vi "DataPacker_MainStateMachine.vi"(0 "DataPacker Queue":refnum<queue>, 1 "DataPacker out":refnum<class "DataPacker.lvclass">, 2 "error IO":errorcluster, 3 "Callers (Main VI name)":string, 6 "MIDAS IP":u32, 8 "MIDAS Sever Port":u16, 10 "Override Max Event size (Data rate bytes/s). Use MIDAS Default = 0":u32) -> (16 "error IO 2":errorcluster)   [LabVIEW 2018, in "feGEM DataPacker.lvlib"]
uses:
  feGEM DataPacker.lvlib
  DataStructures/GEM_BANK_CLUSTER_typedef.ctl
  DataStructures/GEM_DATA_cluster_typedef.ctl
  DataPacker.lvclass
  StateMachineTypeDef.ctl
  GlobalVariables/DataPacker_Global_Stop_Enum.ctl
  DataPacker.lvclass/DataPacker.ctl
  GlobalVariables/DataPacker_Buffer_Usage_Enum.ctl
  GlobalVariables/Set_And_Get_Enum.ctl
  <vilib>/Utility/SystemLogging/NI_SystemLogging.lvlib
panel:
  out "Time since last sleep (ms) 2":dbl(knob) scale=1.0..1000.0
  out "Time Bundling Data (Reading from Queue into LV structures) 2":dbl(knob) scale=0.0..100.0
  out "% Time Packing (Serializing Queued Data) 2":dbl(knob) scale=0.0..100.0
  out "Unsent items in queue (at shutdown)":i32
  out "Frontend Status":string
  out "MIDAS Port":u16
  out "MIDAS Addresss":string
  out "Connection Attempt":u32
  out "MIDAS Reply":string
  out "MIDAS Buffer [for this PC] \nUsage (%)":dbl(knob) scale=0.0..100.0
  out "Log Client info (non fatal)":errorcluster
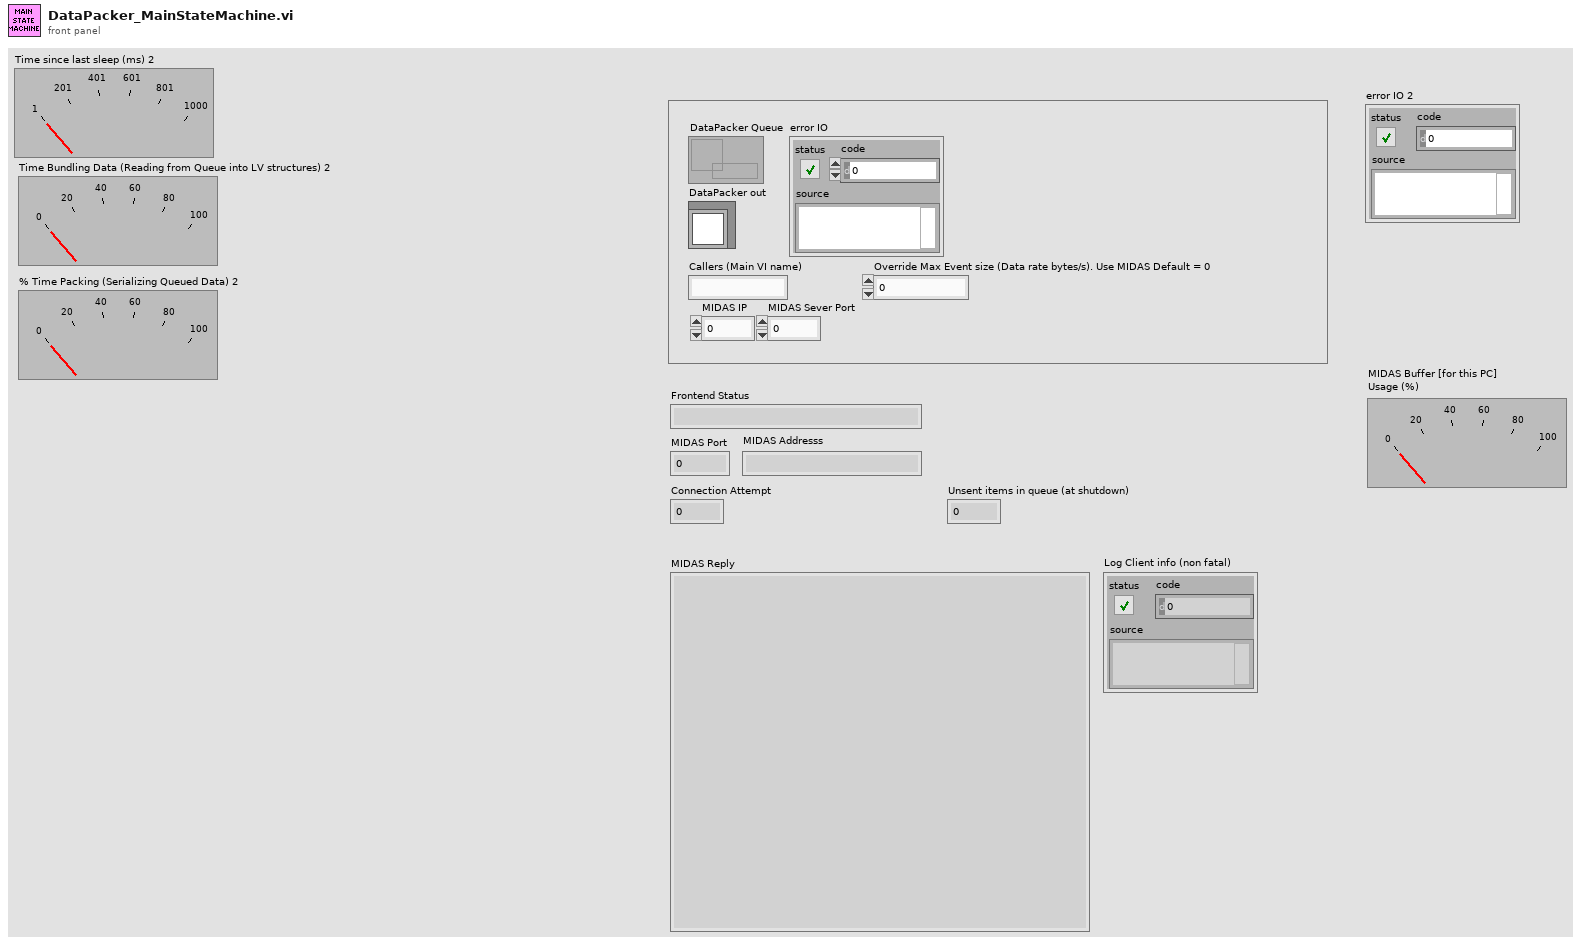
[diagram p1: front panel]
types:
  T1 = typedef "feGEM DataPacker.lvlib/StateMachineTypeDef.ctl" = enum16{"Setup", "Setup SSH", "Connect To Midas", "Get And Set Event Size", "Re-initialise", "Update status", "BundleDataInQueue", "SerializeBundle", "SendData", "Shutdown", "HandleErrorStates", "Wait"}
  T2 = typedef "feGEM DataPacker.lvlib/DataPacker_Global_Stop_Enum.ctl" = enum16{"Reset", "Set Soft Stop", "Get Soft Stop", "Set Hard Stop", "Get Hard Stop", "Get Any Stop"}
  T3 = typedef "feGEM DataPacker.lvlib/DataPacker_Buffer_Usage_Enum.ctl" = enum16{"Get Values", "Set MIDAS Buffer Usage (%)", "Set DataPacker Queue\nUsage (%)"}
  T4 = typedef "feGEM DataPacker.lvlib/Set_And_Get_Enum.ctl" = enum16{"Set", "Get"}
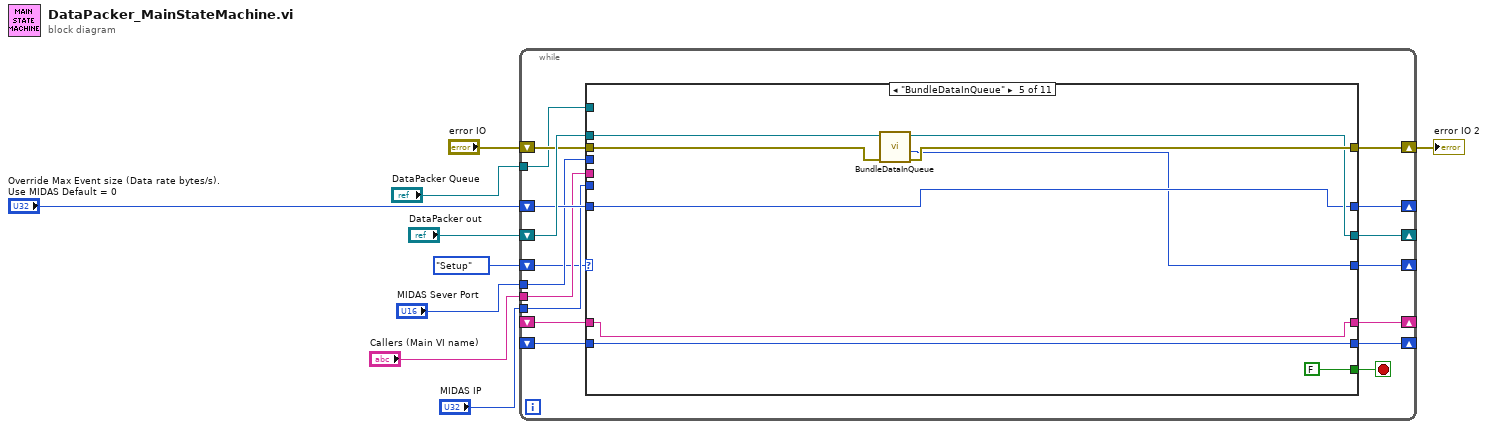
[diagram p0: block diagram]
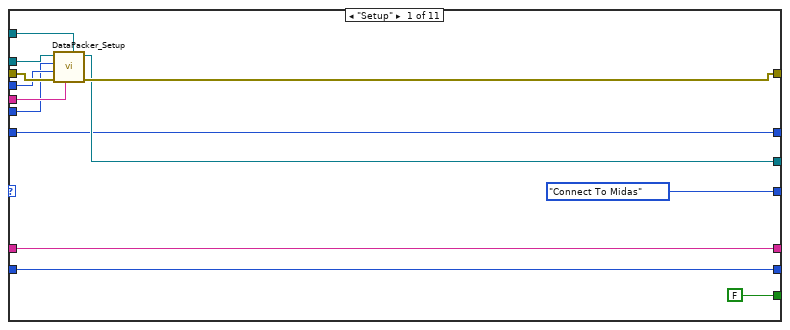
[diagram p2: hidden frame]
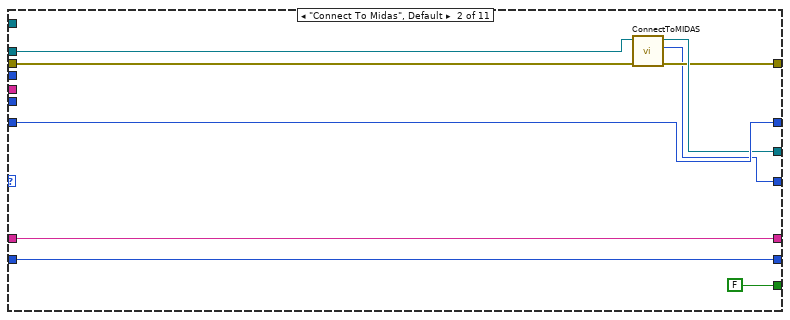
[diagram p3: hidden frame]
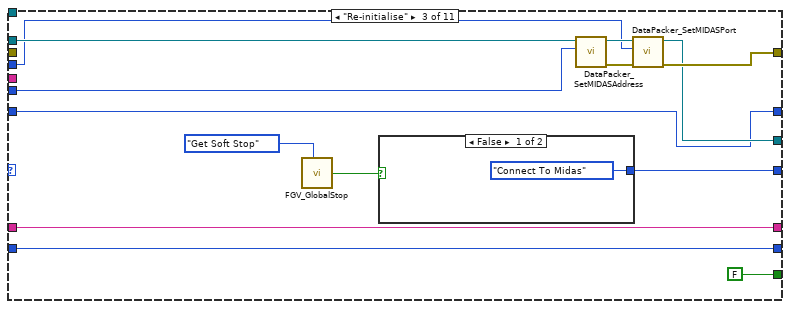
[diagram p4: hidden frame]
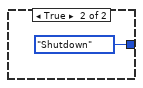
[diagram p5: hidden frame]
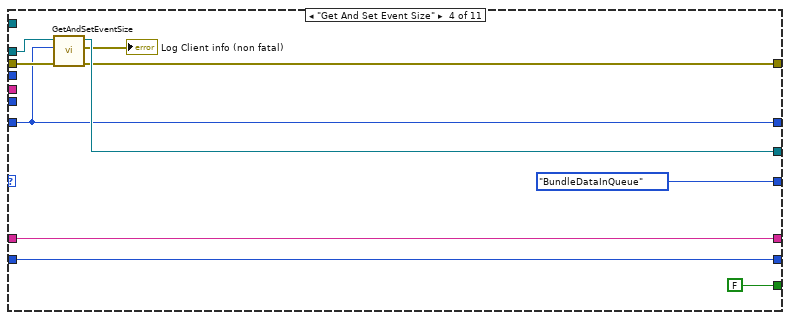
[diagram p6: hidden frame]
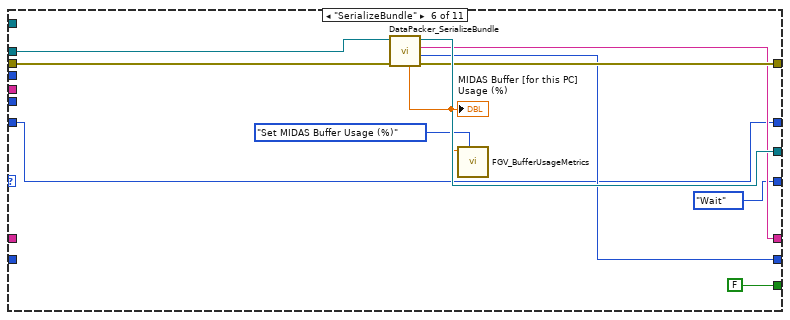
[diagram p7: hidden frame]
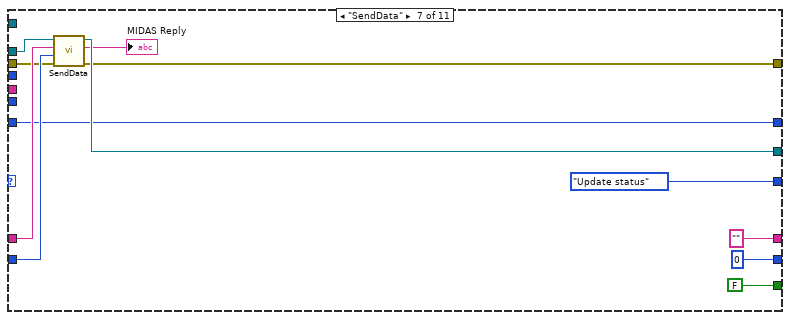
[diagram p8: hidden frame]
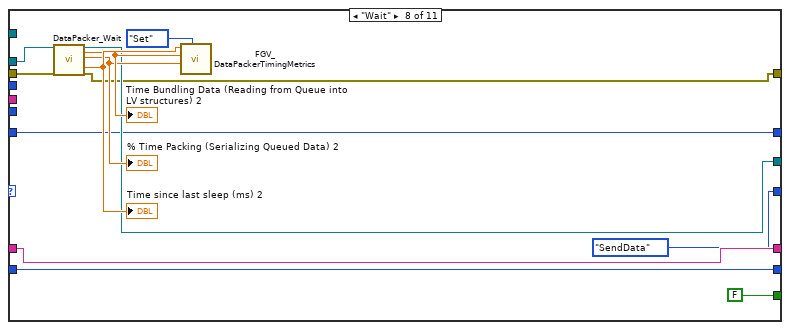
[diagram p9: hidden frame]
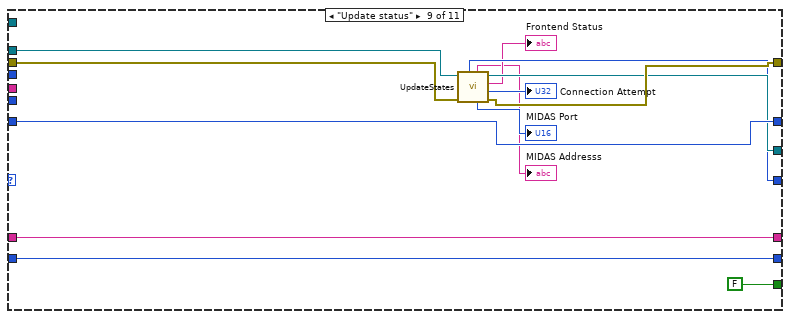
[diagram p10: hidden frame]
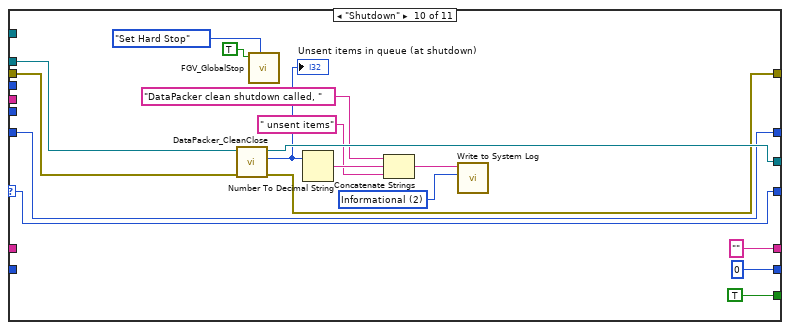
[diagram p11: hidden frame]
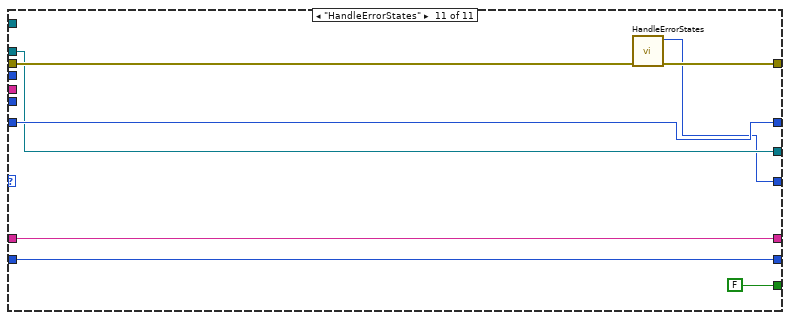
[diagram p12: hidden frame]
diagram:
  n1 = while {
    shift-right: [w10] -> _
    shift-left: StateMachineTypeDef."Setup" ("Enum") -> [w11]
    shift-right: [w24] -> _
    shift-left: "DataPacker out" -> [w26]
    shift-right: [w23] -> w1
    shift-left: "error IO" -> [w25]
    shift-right: [w21] -> _
    shift-left: _ -> [w18]
    shift-right: [w20] -> _
    shift-left: _ -> [w19]
    shift-right: [w17] -> _
    shift-left: "Override Max Event size (Data rate bytes/s). Use MIDAS Default = 0" -> [w22]
    tunnel: "MIDAS Sever Port" -> [w16]
    tunnel: "Callers (Main VI name)" -> [w15]
    tunnel: "DataPacker Queue" -> [w13]
    tunnel: "MIDAS IP" -> [w12]
    stop <- w14 stop-if-true
    n2 = case shown="\"BundleDataInQueue\"" w11 {
      selector: w11 -> [_ _ _ _ _ _ _ _ _ w133 _]
      tunnel: w26 -> [w37 w48 w58 w74 w83 w94 w97 w115 w132 w149 w152]
      tunnel: w25 -> [w39 w47 _ w73 w76 w93 w96 w113 w131 w147 w157]
      tunnel: [w35 w42 w59 w72 w81 w92 w104 w114 w125 w148 w152] -> w24
      tunnel: [w36 w41 w60 w67 w82 w91 w99 w112 w126 w134 w156] -> w23
      tunnel: w22 -> [w33 w44 w53 w68 w77 w87 w100 w109 w127 w143 w155]
      tunnel: [w31 w45 w55 w70 w79 w90 "" w111 w130 "" ("SerialisedData") w153] -> w21
      tunnel: [w32 w43 w54 w69 w80 w89 0 ("Length of \nData bundle") w110 w129 0 ("Length of \nData bundle") w154] -> w20
      tunnel: w19 -> [w32 w43 w54 w69 w80 _ w106 w110 w129 _ w154]
      tunnel: w18 -> [w31 w45 w55 w70 w79 _ w105 w111 w130 _ w153]
      tunnel: [FALSE FALSE FALSE FALSE FALSE FALSE FALSE FALSE FALSE TRUE FALSE] -> w14
      tunnel: [w33 w44 w53 w68 w77 w87 w100 w109 w127 w143 w155] -> w17
      tunnel: w16 -> [w38 _ w57 _ _ _ _ _ _ _ _]
      tunnel: w15 -> [w34 _ _ _ _ _ _ _ _ _ _]
      tunnel: w13 -> [w29 _ _ _ _ _ _ _ _ _ _]
      tunnel: w12 -> [w28 _ w56 _ _ _ _ _ _ _ _]
      tunnel: [StateMachineTypeDef."Connect To Midas" ("Enum") w40 w49 StateMachineTypeDef."BundleDataInQueue" ("Enum") w75 StateMachineTypeDef."Wait" ("Enum") StateMachineTypeDef."Update status" ("Enum") StateMachineTypeDef."SendData" ("Enum") w124 w133 w150] -> w10
      frame "Setup" {
        n3 = call "DataPacker_Setup.vi"("DataPacker Queue"=w29, "Main VI Name"=w34, "error in (no error)"=w39, "Port To Log To"=w38, "Address to Log To"=w28, "DataPacker in"=w37) -> ("error out"=w36:errorcluster, "DataPacker out"=w35:refnum<class "DataPacker.lvclass">)  [unwired: 4 in]
      }
      frame "Connect To Midas", Default {
        n4 = call "ConnectToMIDAS.vi"("error in (no error)"=w47, "DataPacker in"=w48) -> ("error out"=w41:errorcluster, "Enum"=w40:T1, "DataPacker out"=w42:refnum<class "DataPacker.lvclass">)  [unwired: 7 in]
      }
      frame "Re-initialise" {
        n5 = call "FGV_GlobalStop.vi"("Enum"=DataPacker_Global_Stop_Enum."Get Soft Stop") -> ("Stop"=w50:bool)  [unwired: 4 in]
        n6 = case shown="False" w50 {
          tunnel: [StateMachineTypeDef."Connect To Midas" ("Enum") StateMachineTypeDef."Shutdown" ("Enum")] -> w49
          frame False {
          }
          frame True {
          }
        }
        n7 = call "DataPacker_SetMIDASAddress.vi"("Address to Log To"=w56, "DataPacker in"=w58) -> ("error out"=w61:errorcluster, "DataPacker out"=w62:refnum<class "DataPacker.lvclass">)  [unwired: 8 in]
        n8 = call "DataPacker_SetMIDASPort.vi"("error in (no error)"=w61, "Port To Log To"=w57, "DataPacker in"=w62) -> ("error out"=w60:errorcluster, "DataPacker out"=w59:refnum<class "DataPacker.lvclass">)  [unwired: 7 in]
      }
      frame "Get And Set Event Size" {
        n9 = call "GetAndSetEventSize.vi"("error in (no error)"=w73, "Override Max Event size (Data rate bytes/s). Use MIDAS Default = 0"=w68, "DataPacker in"=w74) -> ("error out"=w67:errorcluster, "Log Client info (non fatal)"=→"Log Client info (non fatal)":errorcluster, "DataPacker out"=w72:refnum<class "DataPacker.lvclass">)  [unwired: 6 in]
      }
      frame "BundleDataInQueue" {
        n10 = call "BundleDataInQueue.vi"("error in (no error)"=w76, "DataPacker in"=w83) -> ("error out"=w82:errorcluster, "Enum"=w75:T1, "DataPacker out"=w81:refnum<class "DataPacker.lvclass">)  [unwired: 7 in]
      }
      frame "SerializeBundle" {
        n11 = call "DataPacker_SerializeBundle.vi"("error in (no error)"=w93, "DataPacker in"=w94) -> ("error out"=w91:errorcluster, "Length of \nData bundle"=w89:i32, "SerialisedData"=w90:string, "DataPacker out"=w92:refnum<class "DataPacker.lvclass">, "MIDAS Buffer \n[for this PC] \nUsage (%)"=w86:dbl)  [unwired: 5 in]
        "MIDAS Buffer [for this PC] \nUsage (%)" <- w86
        n12 = call "FGV_BufferUsageMetrics.vi"(7:DataPacker_Buffer_Usage_Enum."Set MIDAS Buffer Usage (%)", "Input"=w86) -> ()  [unwired: 8 in, 2 out]
      }
      frame "SendData" {
        n13 = call "SendData.vi"("error in (no error)"=w96, "Length of \nData bundle"=w106, "SerialisedData"=w105, "DataPacker in"=w97) -> ("error out"=w99:errorcluster, "MIDAS Reply"=→"MIDAS Reply":string, "DataPacker out"=w104:refnum<class "DataPacker.lvclass">)  [unwired: 5 in]
      }
      frame "Wait" {
        n14 = call "DataPacker_Wait.vi"("DataPacker in"=w115, "error in (no error)"=w113) -> ("DataPacker out"=w114:refnum<class "DataPacker.lvclass">, "% Time Bundling Data (Reading from Queue into LV structures)"=w118:dbl, "% Time Packing (Serializing Queued Data)"=w117:dbl, "Time since last sleep(ms)"=w119:dbl, "error out"=w112:errorcluster)  [unwired: 12 in, 1 out]
        "% Time Packing (Serializing Queued Data) 2" <- w117
        "Time Bundling Data (Reading from Queue into LV structures) 2" <- w118
        "Time since last sleep (ms) 2" <- w119
        n15 = call "FGV_DataPackerTimingMetrics.vi"(7:Set_And_Get_Enum."Set", "% Time Packing (Serializing Queued Data)"=w117, "Time Bundling Data (Reading from Queue into LV structures)"=w118, "Time since last sleep (ms)"=w119) -> ()  [unwired: 5 in, 3 out]
      }
      frame "Update status" {
        n16 = call "UpdateStates.vi"("error in (no error)"=w131, "DataPacker in"=w132) -> ("error out"=w126:errorcluster, "Connection Attempt"=→"Connection Attempt":u32, "Frontend Status"=→"Frontend Status":string, "DataPacker out"=w125:refnum<class "DataPacker.lvclass">, "MIDAS Port"=→"MIDAS Port":u16, "MIDAS Addresss"=→"MIDAS Addresss":string, "Enum"=w124:T1)  [unwired: 3 in]
      }
      frame "Shutdown" {
        w142 = 2 items=["Error", "Warning", "Informational"] ("severity")
        n17 = call "DataPacker_CleanClose.vi"("error in (no error)"=w147, "DataPacker in"=w149) -> ("error out"=w134:errorcluster, "Unsent items in queue"=w141:i32, "DataPacker out"=w148:refnum<class "DataPacker.lvclass">)  [unwired: 7 in]
        "Unsent items in queue (at shutdown)" <- w141
        n18 = call "FGV_GlobalStop.vi"("Stop"=TRUE, "Enum"=DataPacker_Global_Stop_Enum."Set Hard Stop") -> ()  [unwired: 3 in, 1 out]
        n19 = Number To Decimal String(number=w141) -> (decimal integer string=w139:string)  [unwired: 1 in]
        n20 = Concatenate Strings("DataPacker clean shutdown called, " ("message"), w139, " unsent items" ("string")) -> (w137:string)
        n21 = call <vilib>:"Write to System Log.vi"("severity"=w142, "message"=w137) -> ()  [unwired: 9 in, 1 out]
      }
      frame "HandleErrorStates" {
        n22 = call "HandleErrorStates.vi"("error in (no error)"=w157) -> ("error out"=w156:errorcluster, "Enum"=w150:T1)  [unwired: 9 in]
      }
    }
  }
  "error IO 2" <- w1
